vi "Test Status String to Enumeration.vi"(11 "Test Status String":string) -> (3 "Channel Status Enumeration":T1)   [LabVIEW 2011]
uses:
  Channel Test Status Enumeration.ctl
panel:
  in  "Channel Status Enumeration for strings output only":T1
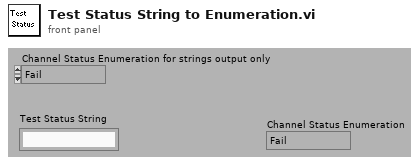
[diagram p1: front panel]
types:
  T1 = typedef "Channel Test Status Enumeration.ctl" = enum16{"Fail", "Pass", "Abort", "Error", "Done", "Pass by Sample", "Fail by Sample", "Pass Override", "Fail Override", "Not Tested"}
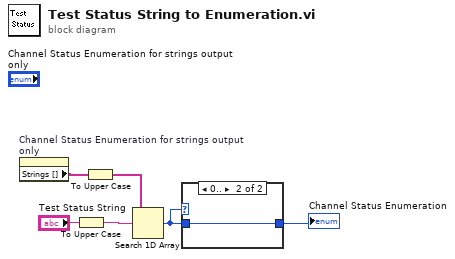
[diagram p0: block diagram]
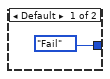
[diagram p2: hidden frame]
diagram:
  n1 = property on="Channel Status Enumeration for strings output only" class="Enum (strict)"() -> ("Strings []"=w5:string[])  [unwired: 2 in, 2 out]
  n2 = To Upper Case(1:"Test Status String") -> (0:w1:string)
  n3 = To Upper Case(1:w5) -> (0:w2:string[])
  n4 = Search 1D Array(1D array=w2, element=w1) -> (index of element=w6:i32)  [unwired: 1 out]
  n5 = case shown="0.." w6 {
    tunnel: w6 -> [_ w8]
    tunnel: [Channel_Test_Status_Enumeration."Fail" ("Channel Status Enumeration") w8] -> w3
    frame Default {
    }
    frame 0.. {
    }
  }
  "Channel Status Enumeration" <- w3
